vi "SetExposureTime.vi"(3 "错误输入":errorcluster, 4 "IMAQdx Session In":T1, 5 "曝光时间/us":u32) -> (0 "错误输出":errorcluster, 1 "IMAQdx Session Out":T1, 2 "ExposureTimeRaw(us)":i64)   [LabVIEW 2012]
uses:
  <vilib>/userDefined/High Color/IMAQdx.ctl
  <resource>/objmgr/imaqdx.rc
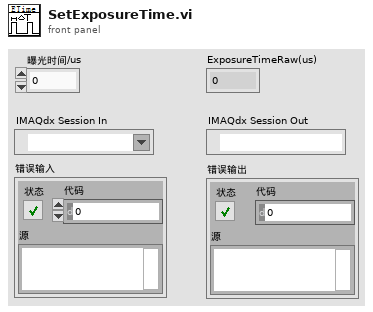
[diagram p1: front panel]
types:
  T1 = typedef "IMAQdx.ctl" = refnum<k21>
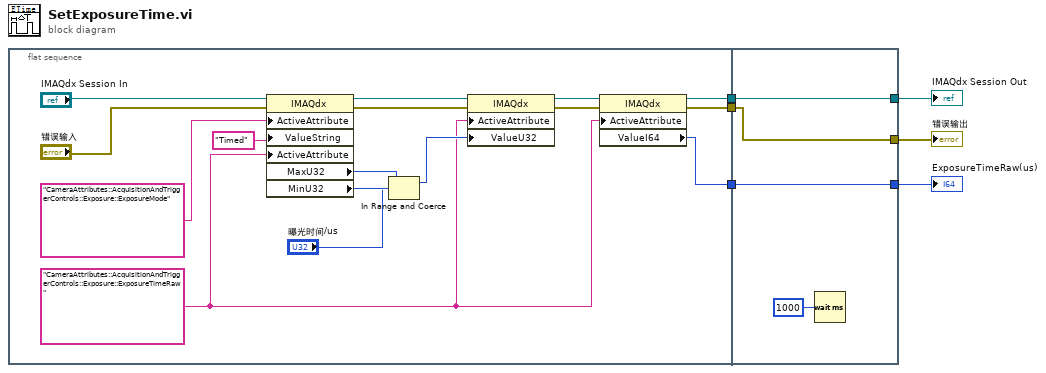
[diagram p0: block diagram]
diagram:
  n1 = flat-sequence {
    tunnel: [w9] -> w6
    tunnel: [w8] -> w4
    tunnel: [w7] -> w2
    tunnel: [w25] -> w5
    tunnel: w6 -> [w25]
    tunnel: w4 -> [w24]
    tunnel: [w24] -> w3
    tunnel: [w23] -> w1
    tunnel: w2 -> [w23]
    frame #0 {
      w10 = "CameraAttributes::AcquisitionAndTriggerControls::Exposure::ExposureTimeRaw" ("ActiveAttribute")
      n2 = property class="IMAQdx"(reference="IMAQdx Session In", error in="错误输入", "ActiveAttribute"="CameraAttributes::AcquisitionAndTriggerControls::Exposure::ExposureMode", "ValueString"="Timed", "ActiveAttribute"=w10) -> (reference out=w18:T1, error out=w17:errorcluster, "MaxU32"=w15:u32, "MinU32"=w16:u32)
      n3 = In Range and Coerce(upper limit=w15, x="曝光时间/us", lower limit=w16) -> (coerced(x)=w13:u32)  [unwired: 1 out]
      n4 = property class="IMAQdx"(reference=w18, error in=w17, "ActiveAttribute"=w10, "ValueU32"=w13) -> (reference out=w12:T1, error out=w11:errorcluster)
      n5 = property class="IMAQdx"(reference=w12, error in=w11, "ActiveAttribute"=w10) -> (reference out=w9:T1, error out=w8:errorcluster, "ValueI64"=w7:i64)
    }
    frame #1 {
      n6 = Wait (ms)(milliseconds to wait=u32 1000 ("等待时间（毫秒）")) -> ()  [unwired: 1 out]
    }
  }
  "IMAQdx Session Out" <- w5
  "错误输出" <- w3
  "ExposureTimeRaw(us)" <- w1
